vi "Read ItemNames.vi"(8 "error in (no error)":errorcluster, 11 "BetterListboxHandle in":refnum<class "BetterListboxHandle.lvclass">) -> (0 "error out":errorcluster, 1 "Number of ItemNames":i32, 2 "Item Names":string[][](array[string]), 3 "BetterListboxHandle out":refnum<class "BetterListboxHandle.lvclass">)   [LabVIEW 2020, in "BetterDragAndDrop.lvlib" / "BetterListboxHandle.lvclass"]
uses:
  BetterListboxHandle.lvclass
  BetterListboxHandle.lvclass/BetterListboxHandle.ctl
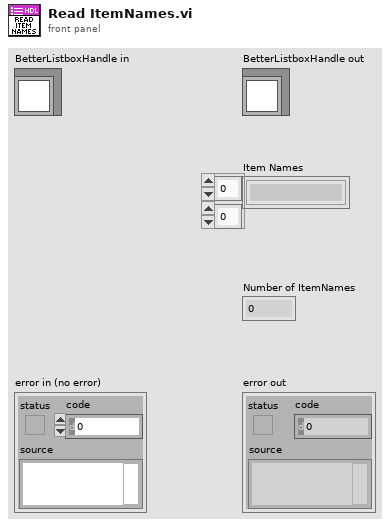
[diagram p1: front panel]
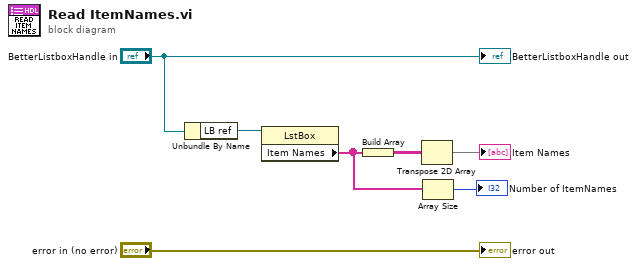
[diagram p0: block diagram]
diagram:
  n1 = Unbundle By Name("BetterListboxHandle in") -> ("LB ref"=w5:refnum<vi>)
  n2 = property class="LstBox"(reference=w5) -> ("Item Names"=w2:string[])  [unwired: 1 in, 2 out]
  n3 = Build Array(w2) -> (w4:string[][])
  n4 = Transpose 2D Array(2D array=w4) -> (transposed array=→"Item Names":string[][])
  n5 = Array Size(array=w2) -> (size(s)=→"Number of ItemNames":i32)
  "error out" <- "error in (no error)"
  "BetterListboxHandle out" <- "BetterListboxHandle in"
